vi "Shoot High Goal State Machine.vi"   [LabVIEW 2013]
uses:
  typedefs/fg_typedef.ctl
  typedefs/singleUseSubstate.ctl
  <vilib>/Rock Robotics/WPI/Solenoid/WPI_SolenoidValue.ctl
  typedefs/subStates.ctl
  <vilib>/Rock Robotics/WPI/Solenoid/WPI_SolenoidGetEnum.vi
panel:
  # "A State Machine to Handle a High Goal Shot"
types:
  T1 = typedef "fg_typedef.ctl" = enum16{"Get", "Set"}
  T2 = enum16{"Shooter Solenoid", "Latch Solenoid", "Right Up Sensor", "Right Down Sensor", "Hold Sensor"}
  T3 = typedef "WPI_SolenoidValue.ctl" = enum16{"Off", "On", "Forward", "Reverse"}
  T4 = typedef "singleUseSubstate.ctl" = enum16{"null", "wait", "shift high", "shift low", "cock shooter", "retract shooter", "latch", "unlatch"}
  T5 = typedef "subStates.ctl" = enum16{"null", "wait", "driver control", "auto", "manual override", "hold position", "rotate", "pickup", "pass", "load", "goto shoot", "shoot high goal", "shoot low goal", "cancel arm", "cancel shooter", "end"}
  T6 = typedef "WPI_DigitalInputDevRef.ctl" = cluster{"DevStatus":errorcluster, "DIO Channel":T7, "Digital Module":T8}
  T7 = typedef "FPGA_DIOChannel.ctl" = enum8{"DIO 1", "DIO 2", "DIO 3", "DIO 4", "DIO 5", "DIO 6", "DIO 7", "DIO 8", "DIO 9", "DIO 10", "DIO 11", "DIO 12", "DIO 13", "DIO 14", "Invalid"}
  T8 = typedef "FPGA_TypedefDigitalModule.ctl" = enum16{"Digital Module 1", "Digital Module 2"}
  T9 = typedef "WPI_SolenoidDevRef.ctl" = cluster{"DevStatus":errorcluster, "Solenoid Module":T10, "Forward Solenoid Channel":T11, "Reverse Solenoid Channel":T11}
  T10 = typedef "FPGA_TypedefSolenoidModule.ctl" = enum16{"Solenoid Module 1", "Solenoid Module 2"}
  T11 = typedef "WPI_SolenoidChannel.ctl" = enum8{"Solenoid 1", "Solenoid 2", "Solenoid 3", "Solenoid 4", "Solenoid 5", "Solenoid 6", "Solenoid 7", "Solenoid 8", "Invalid"}
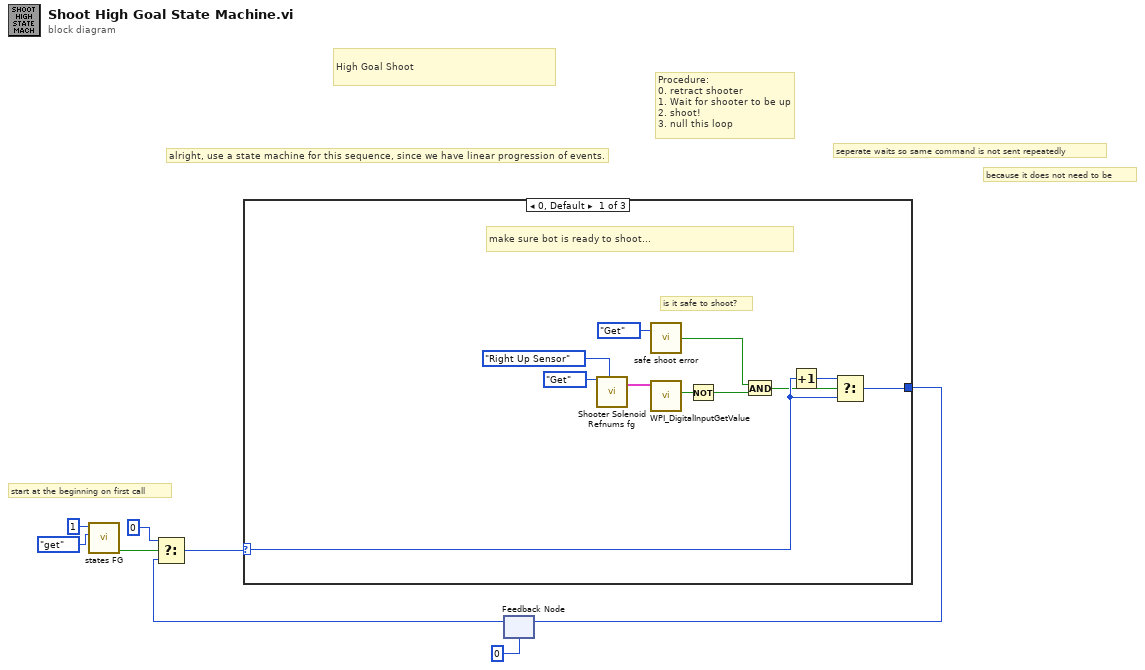
[diagram p0: block diagram]
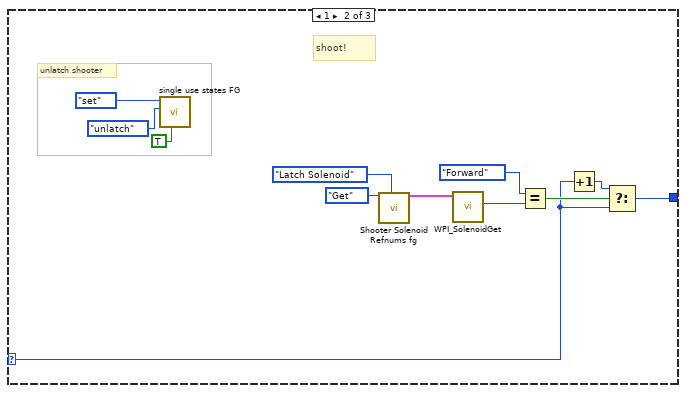
[diagram p2: hidden frame]
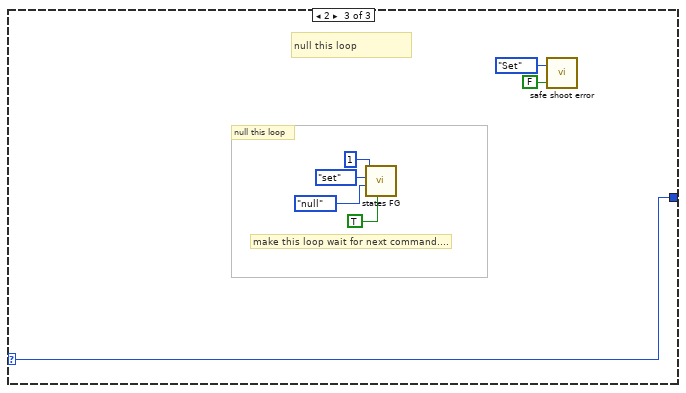
[diagram p3: hidden frame]
diagram:
  # "because it does not need to be"
  # "seperate waits so same command is not sent repeatedly"
  # "start at the beginning on first call"
  # "High Goal Shoot"
  # "Procedure: \n0. retract shooter\n1. Wait for shooter to be up\n2. shoot!\n3. null this loop"
  # "alright, use a state machine for this sequence, since we have linear progression of events."
  n1 = call "states FG.vi"("menu (get)"=enum16{"set", "get"}."get", "Loop ID"=1) -> ("first call?"=w1:bool)  [unwired: 6 in, 3 out]
  n2 = feedback #1(u8 0) -> (w4:u8)
  n3 = Select(t=u8 0, s=w1, f=w4) -> (s? t:f=w3:u8)
  n4 = case shown="0, Default" w3 {
    selector: w3 -> [w16 w21 w38]
    tunnel: [w17 w20 w38] -> w7
    frame 0, Default {
      # "is it safe to shoot?"
      # "make sure bot is ready to shoot..."
      n5 = call "Shooter Solenoid Refnums fg.vi"("Menu"=fg_typedef."Get", "DevRef to Get"=T2."Right Up Sensor") -> ("Selected Sensor"=w13:T6)  [unwired: 15 in, 2 out]
      n6 = call "safe shoot error.vi"("Menu"=fg_typedef."Get") -> ("Can Shoot Safely?"=w11:bool)  [unwired: 1 in]
      n7 = call <vilib>:"WPI_DigitalInputGetValue.vi"("DigitalInputDevRef"=w13) -> ("Value"=w19:bool)  [unwired: 8 in, 2 out]
      n8 = Not(x=w19) -> (.not. x?=w10:bool)
      n9 = And(x=w11, y=w10) -> (x .and. y?=w9:bool)
      n10 = Increment(x=w16) -> (x+1=w18:u8)
      n11 = Select(t=w18, s=w9, f=w16) -> (s? t:f=w17:u8)
    }
    frame 1 {
      # "unlatch shooter"
      # "shoot!"
      n12 = call "single use states FG.vi"("exit in"=TRUE, "substate"=singleUseSubstate."unlatch", "menu (get)"=enum16{"set", "get"}."set") -> ()  [unwired: 5 in, 4 out]
      n13 = call "Shooter Solenoid Refnums fg.vi"("Menu"=fg_typedef."Get", "DevRef to Get"=T2."Latch Solenoid") -> ("Selected Solenoid"=w26:T9)  [unwired: 15 in, 2 out]
      n14 = call-poly <vilib>:"WPI_SolenoidGet.vi"("SolenoidDevRef"=w26) -> ("Value"=w25:T3)  [unwired: 8 in, 2 out]
      n15 = Equal?(x=WPI_SolenoidValue."Forward" ("Value"), y=w25) -> (x = y?=w23:bool)
      n16 = Increment(x=w21) -> (x+1=w22:u8)
      n17 = Select(t=w22, s=w23, f=w21) -> (s? t:f=w20:u8)
    }
    frame 2 {
      # "null this loop"
      # "null this loop"
      # "make this loop wait for next command...."
      n18 = call "states FG.vi"("exit in"=TRUE, "subState in"=subStates."null", "menu (get)"=enum16{"set", "get"}."set", "Loop ID"=1) -> ()  [unwired: 4 in, 4 out]
      n19 = call "safe shoot error.vi"("Can Shoot Safely?"=FALSE, "Menu"=fg_typedef."Set") -> ()  [unwired: 1 out]
    }
  }
  n20 = feedback-in #1(w7) -> ()
